vi "Set Headers2.vi"(0 "handles cluster in":T1 caption="ハンドルクラスター入力", 5 "headers":cluster{"Name":string, "Value":string}[](array[cluster]) caption="ヘッダ", 11 "error in (no error)":errorcluster caption="エラー入力（エラーなし）") -> (4 "handles cluster out":T1 caption="ハンドルクラスター出力", 15 "error out":errorcluster caption="エラー出力")   [LabVIEW 2015]
doc: "Eメールと一緒に送信する補助ヘッダのリストを設定します。実行前にヘッダに指定された値は上書きされます。"
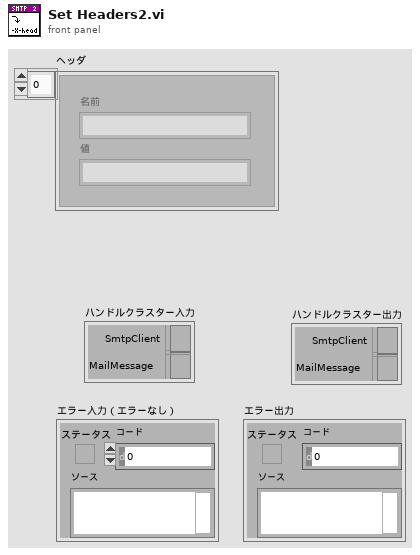
[diagram p1: front panel]
types:
  T1 = cluster{"SmtpClient":refnum<k24>, "MailMessage":refnum<k24>}
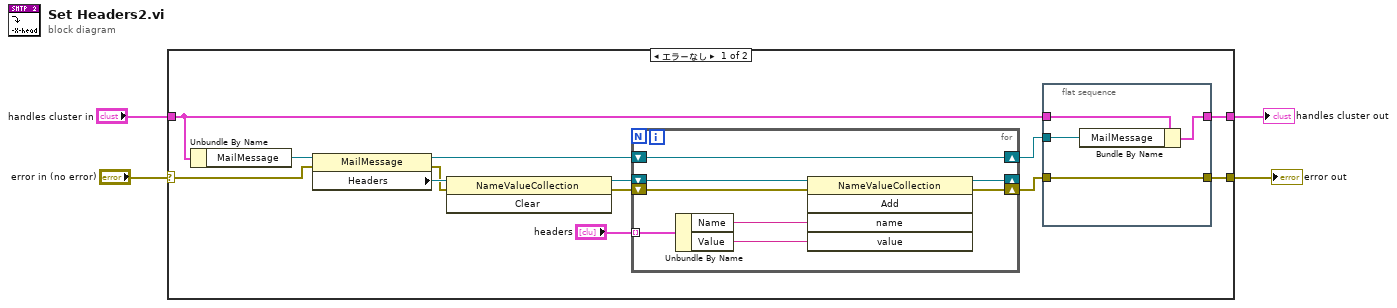
[diagram p0: block diagram]
diagram:
  n1 = case shown="エラーなし" "error in (no error)" {
    selector: "error in (no error)" -> [w13 w31]
    tunnel: [w11 w31] -> w3
    tunnel: "handles cluster in" -> [w17 w30]
    tunnel: [w16 w30] -> w1
    frame No Error {
      n2 = Unbundle By Name(w17) -> ("MailMessage"=w14:refnum<k24>)
      n3 = property class="MailMessage"(reference=w14, error in=w13) -> (reference out=w15:refnum<k24>, error out=w8:errorcluster, "Headers"=w9:refnum<k24>)
      n4 = invoke class="NameValueCollection" method="Clear"(reference=w9, error in=w8) -> (reference out=w7:refnum<k24>, error out=w6:errorcluster)  [unwired: 1 in, 1 out]
      n5 = for {
        shift-right: [w23] -> _
        shift-left: w7 -> [w25]
        shift-right: [w24] -> w10
        shift-left: w6 -> [w21]
        shift-right: [w22] -> w12
        shift-left: w15 -> [w22]
        tunnel: "headers" -> [w20] mode=indexing
        n6 = Unbundle By Name(w20) -> ("Name"=w19:string, "Value"=w18:string)
        n7 = invoke class="NameValueCollection" method="Add"(reference=w25, error in=w21, "name"=w19, "value"=w18) -> (reference out=w23:refnum<k24>, error out=w24:errorcluster)  [unwired: 1 in, 3 out]
      }
      n8 = flat-sequence {
        tunnel: w17 -> [w29]
        tunnel: [w28] -> w16
        tunnel: w12 -> [w27]
        tunnel: [w26] -> w11
        tunnel: w10 -> [w26]
        frame #0 {
          n9 = Bundle By Name(cluster=w29, "MailMessage"=w27) -> (w28:T1)
        }
      }
    }
    frame Error {
    }
  }
  "handles cluster out" <- w1
  "error out" <- w3
